vi "PPAS_AUTOCMD_BEGIN.vi"(9 "Initial Gyo Reading":T3 {"SIN" format="%13.4f"; "COS" format="%13.4f"; "VALUE" format="%13.4f"}, 10 "Robot Starting Pose":T1 {"ROTATION"."SIN" format="%13.4f"; "ROTATION"."COS" format="%13.4f"; "ROTATION"."VALUE" format="%13.4f"; "TRANSLATION"."Y" format="%14.3f"; "TRANSLATION"."X" format="%14.3f"}) -> ()   [LabVIEW 2019]
uses:
  PPAS_AUTOCMD_GLOBALS.vi
  <vilib>/Rock Robotics/WPI/ThirdParty/MJansen/PathPlanner/PathPlanner24.lvlib
  <vilib>/Rock Robotics/WPI/ThirdParty/JAS_Junk/TrajLib/TypeDef/TRANSLATION2D.ctl
  <vilib>/Rock Robotics/WPI/ThirdParty/JAS_Junk/TrajLib/Trajectory_Library.lvlib
  <vilib>/Rock Robotics/WPI/ThirdParty/JAS_Junk/TrajLib/TypeDef/ROTATION2D.ctl
  <vilib>/Rock Robotics/WPI/ThirdParty/JAS_Junk/TrajLib/TypeDef/POSE2D.ctl
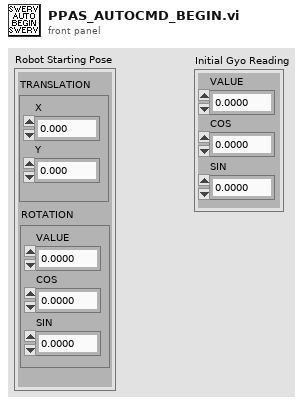
[diagram p1: front panel]
types:
  T1 = typedef "Trajectory_Library.lvlib/POSE2D.ctl" = cluster{"TRANSLATION":T2, "ROTATION":T3}
  T2 = typedef "Trajectory_Library.lvlib/TRANSLATION2D.ctl" = cluster{"X":dbl, "Y":dbl}
  T3 = typedef "Trajectory_Library.lvlib/ROTATION2D.ctl" = cluster{"VALUE":dbl, "COS":dbl, "SIN":dbl}
  T4 = typedef "PathPlanner24.lvlib/PathPlannerCmdPathPlannerAutoConfig.ctl" = cluster{"Command":T5, "ChoreoAuto":bool, "Version":string, "ResetOdom":bool, "Paths":T7[]}
  T5 = typedef "PathPlanner24.lvlib/PathPlannerCommandUtil.ctl" = cluster{"waitTime":dbl, "name":string, "pathName":string, "commands":cluster{"type":T6, "waitTime":dbl, "name":string, "pathName":string}[], "type":T6}
  T6 = typedef "PathPlanner24.lvlib/PathPlanner_CommandUtil_Type_ENUM.ctl" = enum16{"Unknown", "Wait", "Named", "Path", "Sequential", "Parallel", "Race", "Deadline", "PointTowardsZoneEnter", "PointTowardsZoneExit", "TriggerEventStart", "TriggerEventStop", "TriggerEventOneshot"}
  T7 = typedef "PathPlanner24.lvlib/PathPlannerPath.ctl" = cluster{"Reversed":bool, "RotationTargets":T8[], "ConstraintZones":T9[], "EventMarkers":T11[], "GlobalConstraints":T10, "GoalEndState":T12, "AllPoints":T13[], "Name":string, "Waypoints":T14[], "PointTowardsZones":T15[], "IdealStartingState":T16, "IsChoreoPath":bool, "PreventFlipping":bool}
  T8 = typedef "PathPlanner24.lvlib/PathPlannerRotationTarget.ctl" = cluster{"position":dbl, "rotation":T3, "Exists":bool}
  T9 = typedef "PathPlanner24.lvlib/PathPlannerConstraintsZone.ctl" = cluster{"minPosition":dbl, "maxPosition":dbl, "Constraints":T10, "Present":bool}
  T10 = typedef "PathPlanner24.lvlib/PathPlannerPathConstraints.ctl" = cluster{"MaxVelocityMps;":dbl, "MaxAccelerationMpsSq;":dbl, "MaxAngularVelRadPsEc;":dbl, "MaxAngularAccRadPSecSq":dbl, "Exists":bool, "Unlimited":bool, "NominalVoltageVolts":dbl}
  T11 = typedef "PathPlanner24.lvlib/PathPlannerEventMarker.ctl" = cluster{"Position":dbl, "Command":T5, "TriggerName":string, "EndPosition":dbl}
  T12 = typedef "PathPlanner24.lvlib/PathPlannerGoalEndState.ctl" = cluster{"VelocityMPS":dbl, "Rotation":T3}
  T13 = typedef "PathPlanner24.lvlib/PathPlannerPathPoint.ctl" = cluster{"Position":T2, "DistAlongPath":dbl, "MaxV":dbl, "Constraints":T10, "RotationTarget":T8, "WaypointRelativePos":dbl}
  T14 = typedef "PathPlanner24.lvlib/PathPlannerWaypoint.ctl" = cluster{"prevControl":T2, "anchor":T2, "nextControl":T2, "PrevExists":bool, "NextExists":bool}
  T15 = typedef "PathPlanner24.lvlib/PathPlannerPointTowardsZone.ctl" = cluster{"RotationOffset":T3, "Name":string, "TargetPosition":T2, "MinPosition":dbl, "MaxPosition":dbl}
  T16 = typedef "PathPlanner24.lvlib/PathPlannerIdealStartingState.ctl" = cluster{"VelocityMPS":dbl, "Rotation":T3, "NotNull":bool}
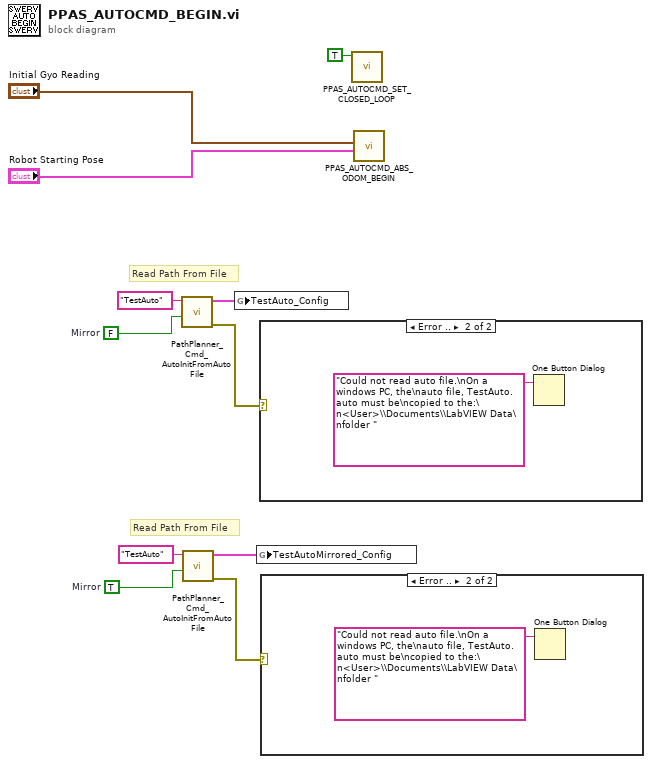
[diagram p0: block diagram]
diagram:
  w1 = TRUE  # Mirror
  w5 = FALSE  # Mirror
  # "Read Path From File"
  # "Read Path From File"
  n1 = call <vilib>:"PathPlanner_Cmd_AutoInitFromAutoFile.vi"("Mirror"=w5, "FileName"="TestAuto") -> ("error out"=w8:errorcluster, "PathPlanner_Cmd_AutoConfig"=w7:T4)  [unwired: 6 in, 2 out]
  n2 = call <vilib>:"PathPlanner_Cmd_AutoInitFromAutoFile.vi"("Mirror"=w1, "FileName"="TestAuto") -> ("error out"=w3:errorcluster, "PathPlanner_Cmd_AutoConfig"=w2:T4)  [unwired: 6 in, 2 out]
  n3 = global write "PPAS_AUTOCMD_GLOBALS.vi" "TestAuto_Config"(w7) -> ()
  n4 = global write "PPAS_AUTOCMD_GLOBALS.vi" "TestAutoMirrored_Config"(w2) -> ()
  n5 = case shown="Error .." w8 {
    frame No Error {
    }
    frame Error {
      n6 = One Button Dialog(message="Could not read auto file.\nOn a windows PC, the\nauto file, TestAuto.auto must be\ncopied to the:\n<User>\\Documents\\LabVIEW Data\nfolder ") -> ()  [unwired: 1 in, 1 out]
    }
  }
  n7 = case shown="Error .." w3 {
    frame No Error {
    }
    frame Error {
      n8 = One Button Dialog(message="Could not read auto file.\nOn a windows PC, the\nauto file, TestAuto.auto must be\ncopied to the:\n<User>\\Documents\\LabVIEW Data\nfolder ") -> ()  [unwired: 1 in, 1 out]
    }
  }
  n9 = call "PPAS_AUTOCMD_SET_CLOSED_LOOP.vi"("AUTO_CLOSED_LOOP"=TRUE) -> ()  [unwired: 11 in]
  n10 = call "PPAS_AUTOCMD_ABS_ODOM_BEGIN.vi"("Initial Pose"="Robot Starting Pose", "Initial Gyro Angle"="Initial Gyo Reading") -> ()  [unwired: 9 in, 1 out]
